vi "Autosampler Shake Tray.vi"(7 "Correlation ID":u32, 8 "error in (no error)":errorcluster, 11 "Application in":refnum<class "Application.lvclass">) -> (0 "error out":errorcluster, 3 "Application out":refnum<class "Application.lvclass">)   [LabVIEW 2023, in "Application.lvlib" / "Application.lvclass"]
uses:
  Application.lvclass
  Application.lvclass/Application.ctl
  <vilib>/ActorFramework/Message Enqueuer/Message Enqueuer.lvclass/Message Enqueuer.ctl
  <vilib>/ActorFramework/Message Enqueuer/Enqueue.vi
  Hardware/Autosampler Messages/Shake Tray Msg/Shake Tray Msg.lvclass
  C:/Program Files/National Instruments/LabVIEW 2023/vi.lib/ActorFramework/Message/Message.lvclass
  <vilib>/ActorFramework/Message Priority Queue/Priority Enqueue.vi
  Hardware/Device Messages/Save CorrID Msg/Save CorrID Msg.lvclass
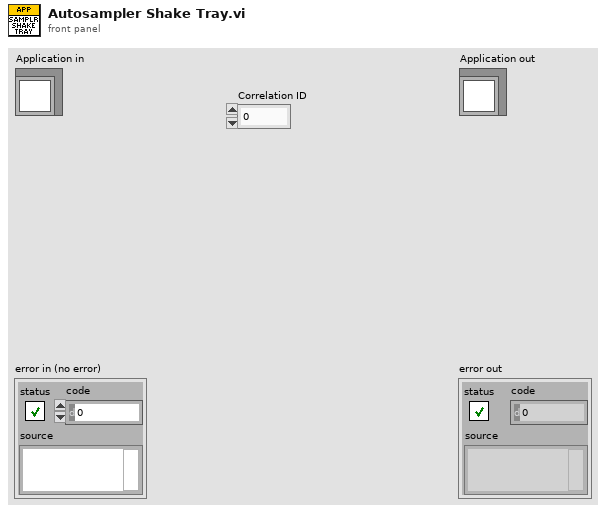
[diagram p1: front panel]
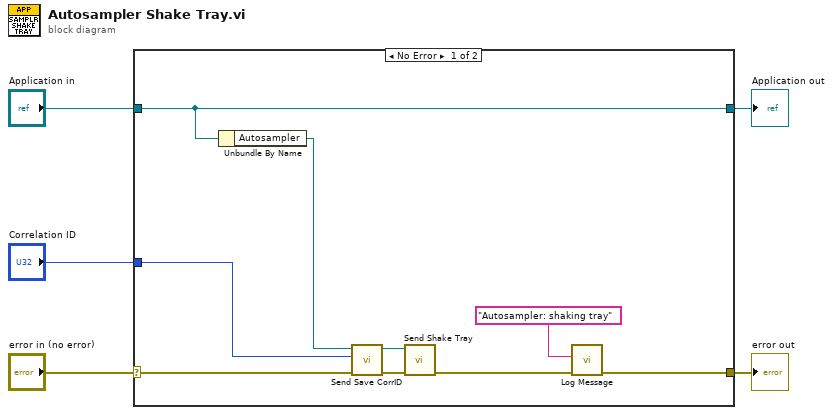
[diagram p0: block diagram]
diagram:
  n1 = case shown="No Error" "error in (no error)" {
    selector: "error in (no error)" -> [w10 w16]
    tunnel: [w13 w16] -> w4
    tunnel: [w14 w15] -> w2
    tunnel: "Application in" -> [w14 w15]
    tunnel: "Correlation ID" -> [w6 _]
    frame No Error {
      n2 = Unbundle By Name(w14) -> ("Autosampler"=w7:refnum<class "Message Enqueuer.lvclass">)
      n3 = call "Send Save CorrID.vi"("error in (no error)"=w10, "Correlation ID"=w6, "Message Enqueuer"=w7) -> ("error out"=w9:errorcluster, "Message Enqueuer out"=w8:refnum<class "Message Enqueuer.lvclass">)  [unwired: 7 in]
      n4 = call "Send Shake Tray.vi"("error in (no error)"=w9, "Message Enqueuer"=w8) -> ("error out"=w12:errorcluster)  [unwired: 8 in, 1 out]
      n5 = call "Log Message.vi"("error constant"=w12, "input"="Autosampler: shaking tray" ("format string")) -> ("error constant 2"=w13:errorcluster)  [unwired: 8 in, 1 out]
    }
    frame Error {
    }
  }
  "error out" <- w4
  "Application out" <- w2
